vi "Color Steps Control.vi"(7 "Calling VI Ref":refnum<vi>) -> ()   [LabVIEW 2020]
uses:
  <vilib>/Utility/miscctls.llb/LVPointTypeDef.ctl
  Color Steps Type Def/Color Steps Presets Type.ctl
  Color Steps Type Def/Color Steps Step Type.ctl
  Laser Control/Laser Power Control/Laser Power Control Type Defs/Laser Power Ctrl Base Type.ctl
  Color Steps Type Def/Color Steps Notifier Type.ctl
  Color Steps Type Def/Color Step Actions.ctl
  Hardware Configuration/Hardware Configuration Controls/Device Type.ctl
  Hardware Configuration/Hardware Configuration Controls/Device Function.ctl
  Laser Control/Laser Power Control/Laser Power Control Type Defs/Laser Power Ctrl Messenger Actions.ctl
  Device Library/Spinning Disk/Spinning Disk Polymorphic Messenger/Status.vi
  Device Library/Filter Wheels/Polymorphic Filter Wheel Messenger/FW Get Position.vi
  Device Library/Spinning Disk/Spinning Disk Polymorphic Messenger/Set Dichroic Position.vi
  Device Library/Spinning Disk/Spinning Disk Polymorphic Messenger/Set Filter Position.vi
  Device Library/Filter Wheels/Polymorphic Filter Wheel Messenger/FW Set Position.vi
panel:
  in  "Tab Control":enum32{"Step Control", "Setup"}(tab)
  in  "Presets":u16(ring) items=["None"]
  in  "Step":T1(radio)
  in  "Add Step":bool
  in  "Update Step":bool
  in  "Remove Step":bool
  in  "Clear All":bool
  in  "Preset_Name":string
  in  "Step_Name_01":string
  in  "Step_Name_02":string
  in  "Step_Name_03":string
  in  "Step_Name_04":string
  in  "Step_Name_05":string
  in  "Save Preset":bool
  in  "Setup":bool=TRUE
  in  "Quit":bool
  # "Preset Name:"
  # "Step 01 Name:"
  # "Step 04 Name:"
  # "Step 02 Name:"
  # "Step 05 Name:"
  # "Step 03 Name:"
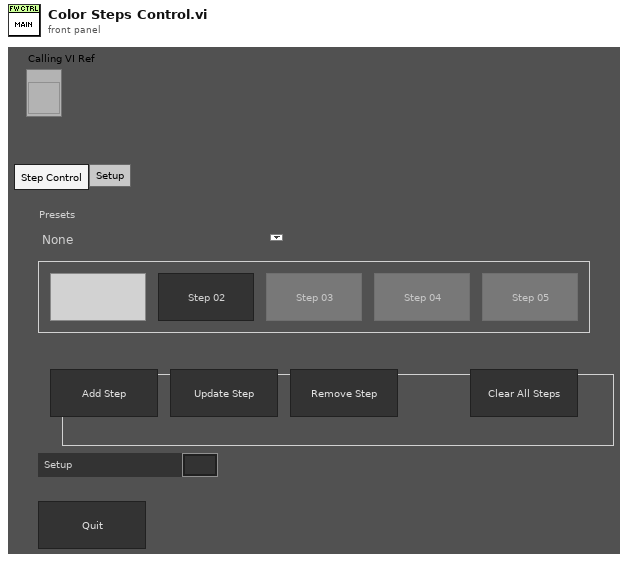
[diagram p1: front panel]
types:
  T1 = enum32{"Step 01", "Step 02", "Step 03", "Step 04", "Step 05"}
  T2 = typedef "Device Function.ctl" = enum16{"Primary", "Secondary", "Overview", "Wide Field Drift Correction", "642 nm Excitation", "560 nm Excitation", "940 nm Excitation", "546 nm Excitation", "488 nm Excitation", "405 nm Excitation", "Objective Drift Correction", "4Pi Objective Lock", "Objective XY", "Objective Z", "Sample XY", "Sample Coarse Z", "Sample Z", "4Pi Lower", "4Pi Upper", "Mojo", "Adj Cavity", "Line Scanning", "Alert"}
  T3 = typedef "Device Type.ctl" = enum16{"AOTF", "Camera", "Deformable Mirror", "Laser", "Microscope Base", "Shutter", "Stage", "Waveform", "FPGA", "Email", "Filter Wheel", "Spinning Disk"}
  T4 = typedef "Color Steps Notifier Type.ctl" = cluster{"Actions":T5, "Set Step":i32, "Current Step":i32, "Last Step?":bool, "Received?":bool, "Preset Index":i32}
  T5 = typedef "Color Step Actions.ctl" = enum16{"Add Step", "Update Step", "Remove Step", "Clear All", "Get Status", "Next Step", "Go To Step", "Save Preset", "Change Preset", "Update Names", "Quit"}
  T6 = typedef "Color Steps Presets Type.ctl" = cluster{"Preset Name":string, "Steps":T7[]}
  T7 = typedef "Color Steps Step Type.ctl" = cluster{"Power Ctrl":T8[], "Filter Wheel Position":i32, "Step Name":string, "Wavelengths":u16[], "SD Dichroic":i32, "SD Filter Wheel":i32}
  T8 = typedef "Laser Power Ctrl Base Type.ctl" = cluster{"Active":bool, "Power":dbl, "Ctrl Mode":u16}
  T9 = enum16{"Always On", "Always Off", "Off While Running"}
  T10 = typedef "LVPointTypeDef.ctl" = cluster{"Horizontal":i16, "Vertical":i16}
  T11 = enum8{"Enabled", "Disabled", "Disabled and Grayed Out"}
  T12 = typedef "LVRectTypeDef.ctl" = cluster{"Left":i16, "Top":i16, "Right":i16, "Bottom":i16}
  T13 = typedef "LVBoundsTypeDef.ctl" = cluster{"Width":u32, "Height":u32}
  T14 = typedef "Laser Power Ctrl Messenger Actions.ctl" = enum16{"All Active On", "All Off", "Adjust Power", "Line On/Off", "Get Status"}
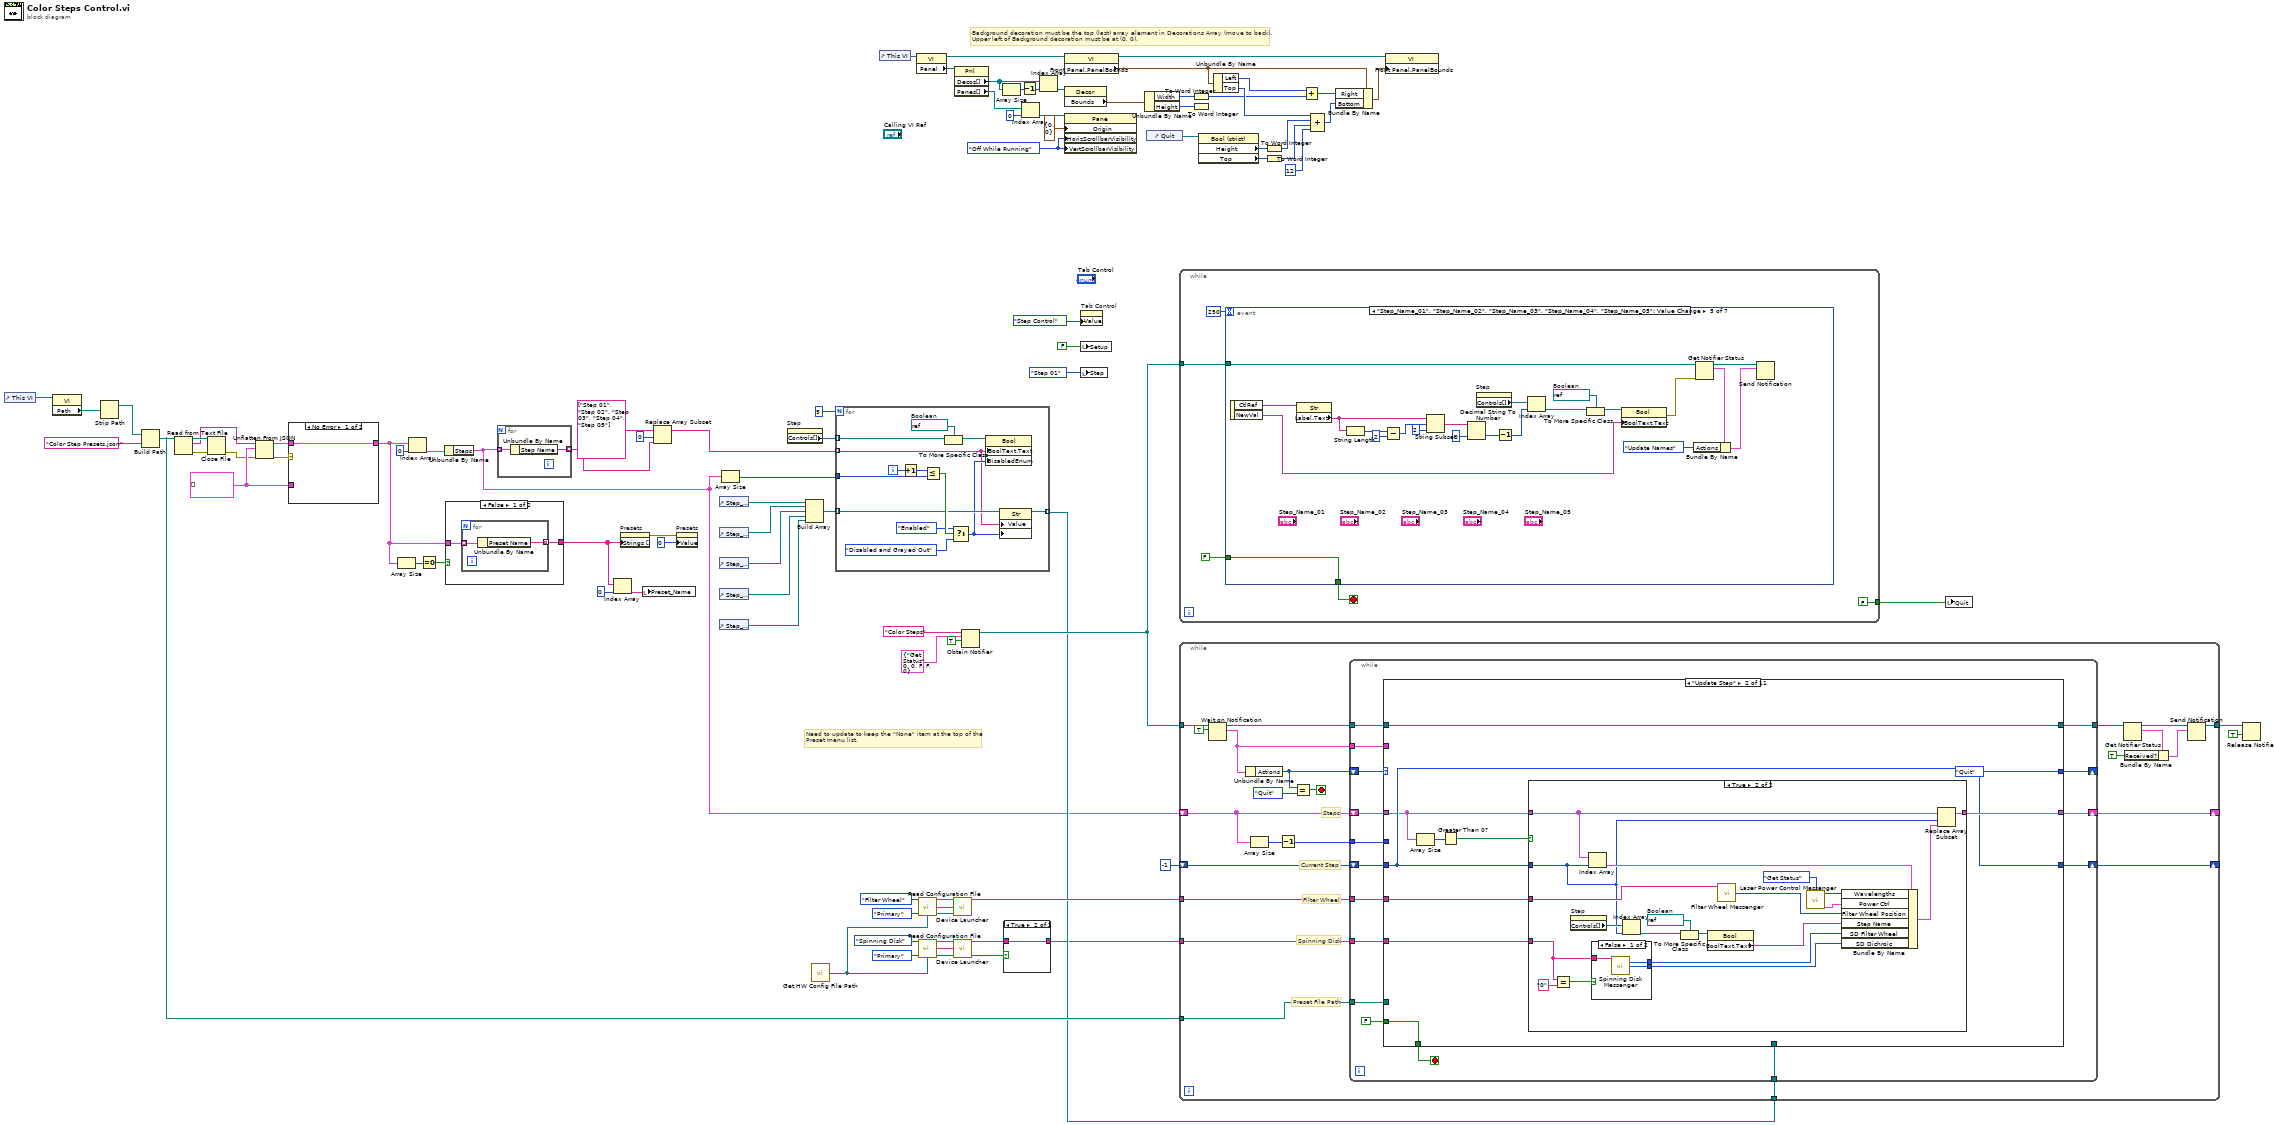
[diagram p0: block diagram]
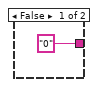
[diagram p2: hidden frame]
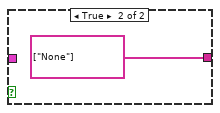
[diagram p3: hidden frame]
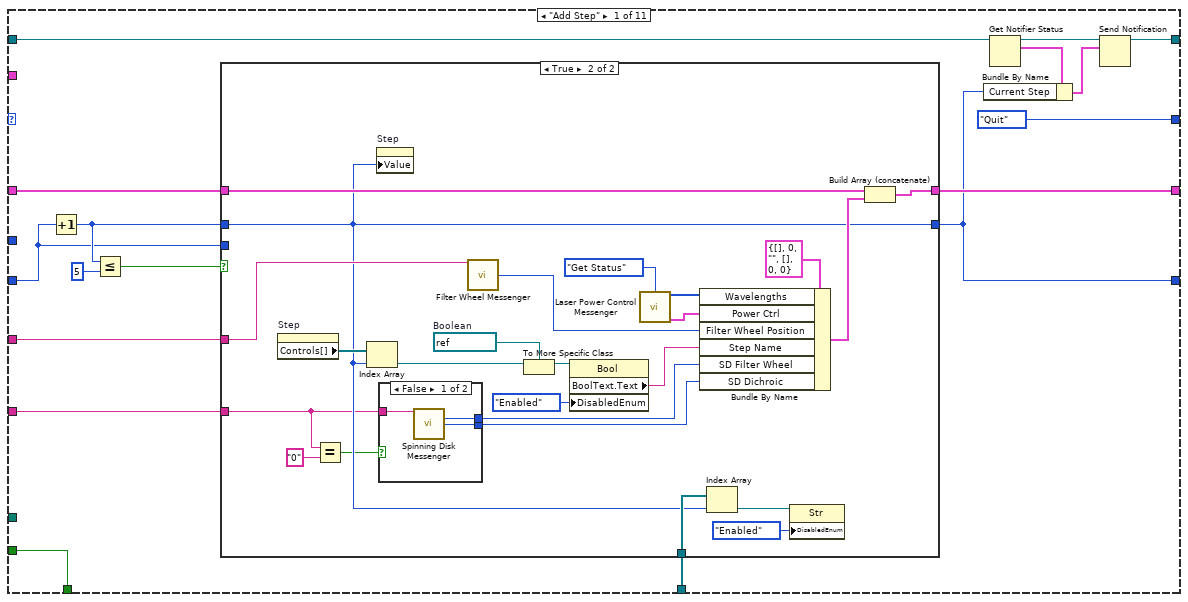
[diagram p4: hidden frame]
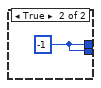
[diagram p6: hidden frame]
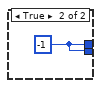
[diagram p8: hidden frame]
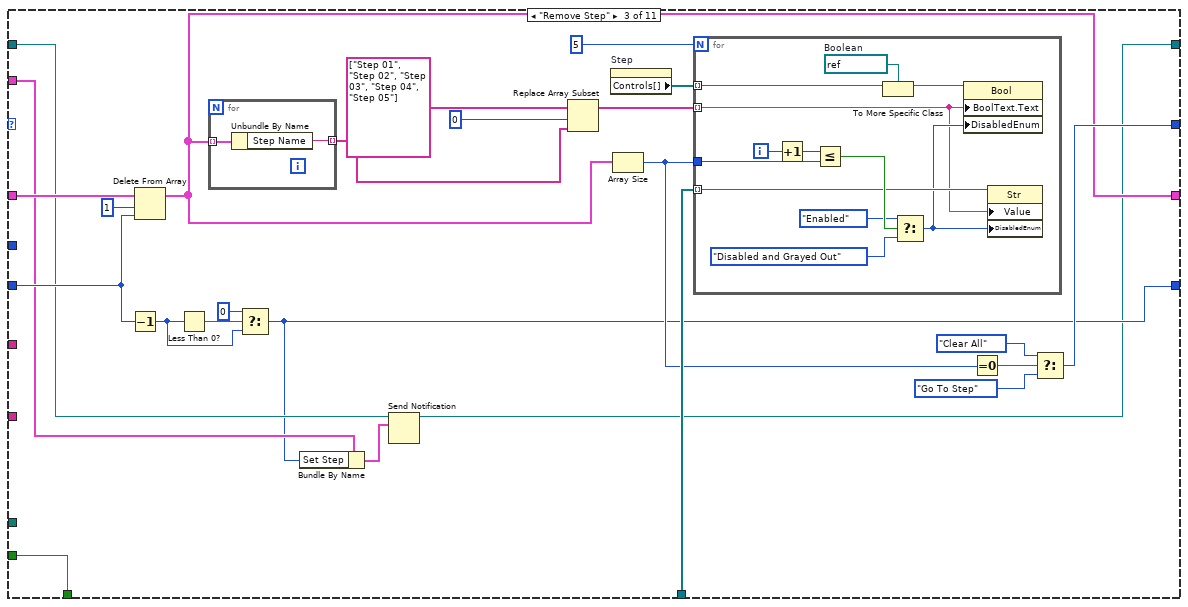
[diagram p9: hidden frame]
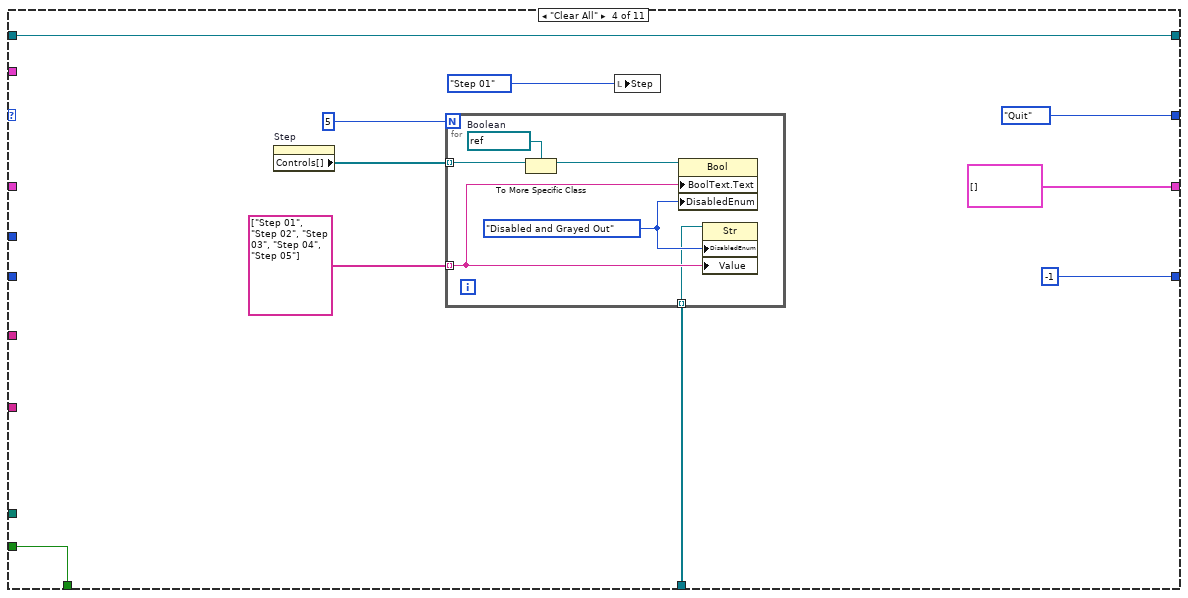
[diagram p10: hidden frame]
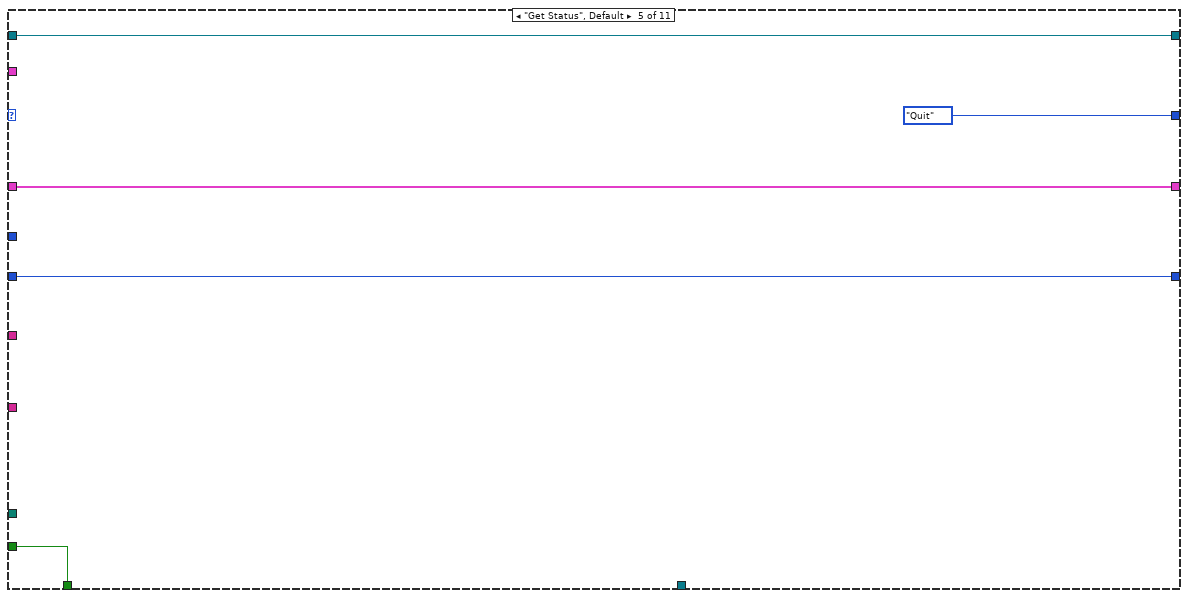
[diagram p11: hidden frame]
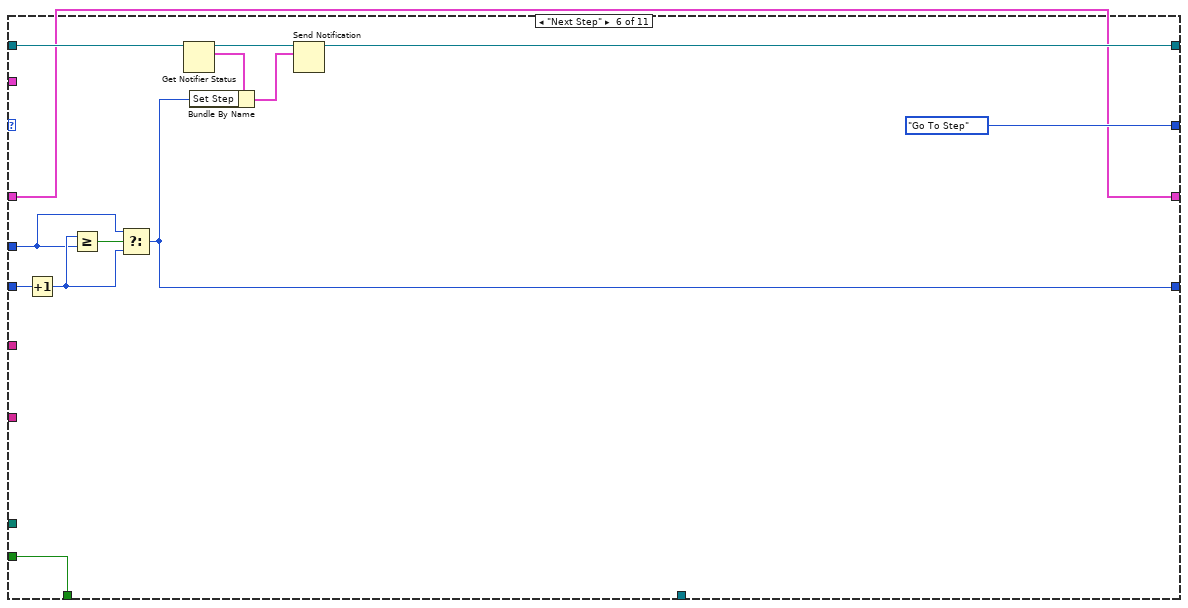
[diagram p12: hidden frame]
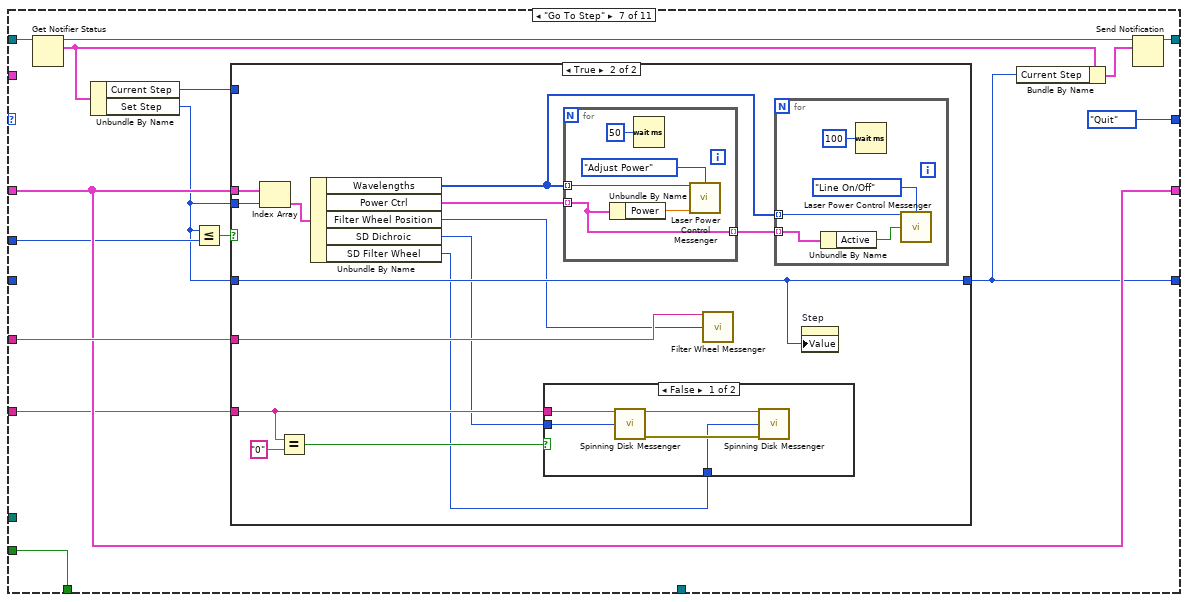
[diagram p13: hidden frame]
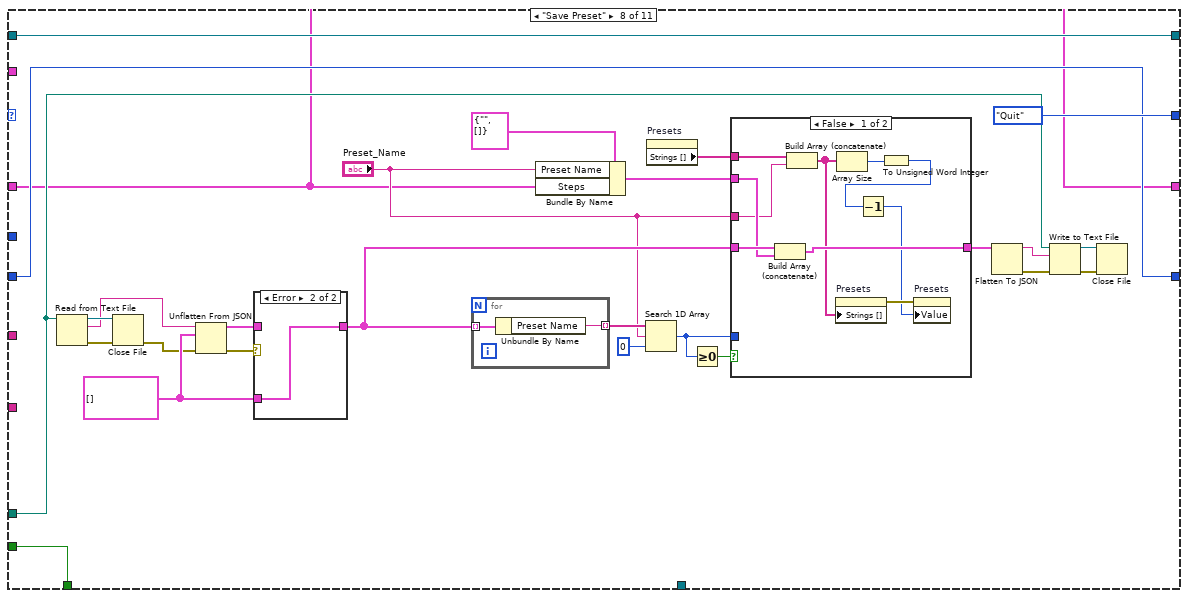
[diagram p16: hidden frame]
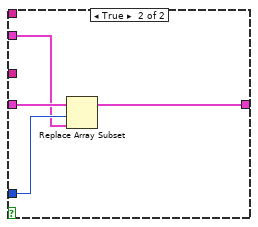
[diagram p17: hidden frame]
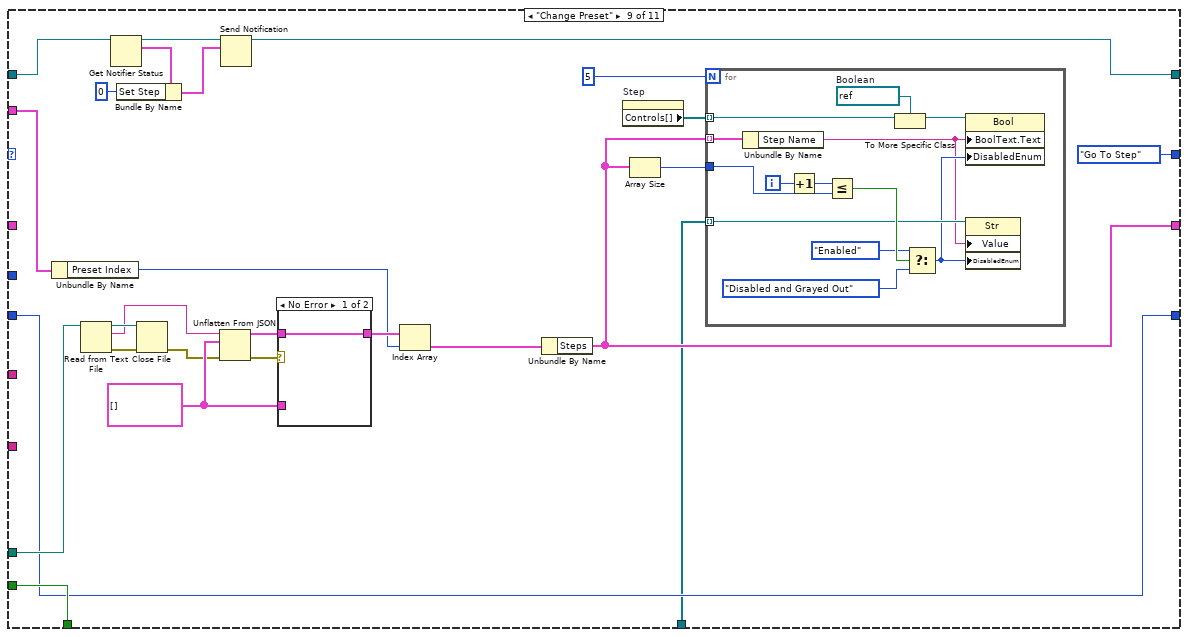
[diagram p19: hidden frame]
diagram:
  w48 = T6[] []
  w75 = T9."Off While Running" ("Vertical Scrollbar Visibility")
  # "Need to update to keep the \"None\" item at the top of the\nPreset menu list."
  # "Background decoration must be the top (last) array element in Decorations Array (move to back).\nUpper left of Background decoration must be at (0, 0)."
  n1 = control-ref of="This VI"() -> (w63:refnum<vi>)
  n2 = property class="VI"(reference=w63) -> ("Path"=w62:path)  [unwired: 1 in, 2 out]
  n3 = Strip Path(path=w62) -> (stripped path=w58:path)  [unwired: 1 out]
  n4 = Build Path(base path=w58, name or relative path="Color Step Presets.json") -> (appended path=w22:path)
  n5 = Read from Text File(file (use dialog)=w22) -> (refnum out=w47:refnum<file>, text=w44:string, error out=w46:errorcluster)  [unwired: 3 in, 1 out]
  n6 = Close File(refnum=w47, error in=w46) -> (error out=w45:errorcluster)  [unwired: 1 out]
  n7 = Unflatten From JSON(JSON string=w44, type and defaults=w48, error in (no error)=w45) -> (value=w59:T6[], error out=w60:errorcluster)  [unwired: 4 in]
  n8 = case shown="No Error" w60 {
    tunnel: w59 -> [w93 _]
    tunnel: w48 -> [_ w94]
    tunnel: [w93 w94] -> w18
    frame No Error {
    }
    frame Error {
    }
  }
  n9 = Array Size(array=w18) -> (size(s)=w17:i32)
  n10 = Index Array(array=w18, index=0) -> (element=w31:T6)
  n11 = Equal To 0?(x=w17) -> (x = 0?=w16:bool)
  n12 = Unbundle By Name(w31) -> ("Steps"=w12:T7[])
  n13 = case shown="False" w16 {
    tunnel: w18 -> [w96 _]
    tunnel: [w95 string[] ["None"]] -> w20
    frame False {
      n14 = for {
        tunnel: w96 -> [w98] mode=indexing
        tunnel: [w97] -> w95 mode=indexing
        n15 = Unbundle By Name(w98) -> ("Preset Name"=w97:string)
      }
    }
    frame True {
    }
  }
  n16 = for {
    tunnel: w12 -> [w101] mode=indexing
    tunnel: [w100] -> w13 mode=indexing
    n17 = Unbundle By Name(w101) -> ("Step Name"=w100:string)
  }
  n18 = Index Array(array=w20, index=0) -> (element=w29:string)
  n19 = property on="Presets" class="Ring (strict)"("Strings []"=w20) -> (error out=w42:errorcluster)  [unwired: 2 in, 1 out]
  n20 = local write "Preset_Name"(w29) -> ()
  n21 = Replace Array Subset(array=string[] ["Step 01", "Step 02", "Step 03", "Step 04", "Step 05"], new element=w13, index=0) -> (w11:string[])
  n22 = property on="Presets" class="Ring (strict)"(error in=w42, "Value"=u16 0) -> ()  [unwired: 1 in, 2 out]
  n23 = control-ref of="Step_Name_01"() -> (w57:refnum<vi>)
  n24 = control-ref of="Step_Name_02"() -> (w53:refnum<vi>)
  n25 = control-ref of="Step_Name_03"() -> (w54:refnum<vi>)
  n26 = control-ref of="Step_Name_04"() -> (w55:refnum<vi>)
  n27 = control-ref of="Step_Name_05"() -> (w56:refnum<vi>)
  n28 = Array Size(array=w12) -> (size(s)=w40:i32)
  n29 = property on="Step" class="RadioBtnsControl (strict)"() -> ("Controls[]"=w51:refnum<vi>[])  [unwired: 2 in, 2 out]
  n30 = Build Array(w57, w53, w54, w55, w56) -> (w43:refnum<vi>[])
  n31 = call "Get HW Config File Path.vi"() -> ("File Path"=w4:path)  [unwired: 14 in, 1 out]
  n32 = for {
    N: 5 -> [_]
    tunnel: [w114] -> w21 mode=indexing
    tunnel: w51 -> [w113] mode=indexing
    tunnel: w43 -> [w105] mode=indexing
    tunnel: w40 -> [w104]
    tunnel: w11 -> [w102] mode=indexing
    i -> [w110]
    w112 = refnum<vi> refnum  # Boolean
    n33 = Increment(x=w110) -> (x+1=w109:i32)
    n34 = Less Or Equal?(x=w109, y=w104) -> (x <= y?=w108:bool)
    n35 = To More Specific Class(target class=w112, reference=w113) -> (specific class reference=w111:refnum<vi>)  [unwired: 1 in, 1 out]
    n36 = Select(t=T11."Enabled" ("Disabled"), s=w108, f=T11."Disabled and Grayed Out") -> (s? t:f=w103:T11)
    n37 = property class="Bool"(reference=w111, "BoolText.Text"=w102, "DisabledEnum"=w103) -> ()  [unwired: 1 in, 2 out]
    n38 = property class="Str"(reference=w105, "Value"=w102, "DisabledEnum"=w103) -> (reference out=w114:refnum<vi>)  [unwired: 1 in, 1 out]
  }
  n39 = control-ref of="This VI"() -> (w67:refnum<vi>)
  n40 = property class="VI"(reference=w67) -> (reference out=w76:refnum<vi>, "Panel"=w68:refnum<vi>)  [unwired: 1 in, 1 out]
  n41 = call "Read Configuration File.vi"("Device Type"=Device_Type."Filter Wheel", "Device Function"=Device_Function."Primary", "Config File Path"=w4) -> ("Unique Notifier Name"=w28:string, "Device Ports/IDs/Channels"=w26:string[], "Device Engine Path"=w27:path)  [unwired: 9 in, 1 out]
  n42 = call "Read Configuration File.vi"("Device Type"=Device_Type."Spinning Disk", "Device Function"=Device_Function."Primary", "Config File Path"=w4) -> ("Unique Notifier Name"=w5:string, "Device Ports/IDs/Channels"=w7:string[], "Device Engine Path"=w6:path)  [unwired: 9 in, 1 out]
  n43 = call "Device Launcher.vi"("Notifier Name"=w28, "Device Ports/IDs/Channels"=w26, "Device Engine Path"=w27) -> ("Notifier Name"=w23:string)  [unwired: 11 in, 1 out]
  n44 = call "Device Launcher.vi"("Notifier Name"=w5, "Device Ports/IDs/Channels"=w7, "Device Engine Path"=w6) -> ("Notifier Name"=w2:string, "Running?"=w3:bool)  [unwired: 11 in]
  n45 = property class="Pnl"(reference=w68) -> ("Decos[]"=w66:refnum<vi>[], "Panes[]"=w72:refnum<vi>[])  [unwired: 1 in, 2 out]
  n46 = Obtain Notifier(name (unnamed)="Color Steps", notification data type=T4 {"Actions"=enum."Get Status", "Set Step"=0, "Current Step"=0, "Last Step?"=FALSE, "Received?"=FALSE, "Preset Index"=0} ("Color Steps Note Type"), create if not found? (T)=TRUE) -> (notifier out=w35:refnum<notifier>)  [unwired: 1 in, 2 out]
  n47 = Array Size(array=w66) -> (size(s)=w64:i32)
  n48 = case shown="True" w3 {
    tunnel: w2 -> [_ w116]
    tunnel: ["0" w116] -> w1
    frame False {
    }
    frame True {
    }
  }
  n49 = Decrement(x=w64) -> (x-1=w65:i32)
  n50 = Index Array(array=w72, index=0) -> (element=w71:refnum<vi>)
  n51 = Index Array(array=w66, index=w65) -> (element=w74:refnum<vi>)
  n52 = property class="VI"(reference=w76) -> (reference out=w78:refnum<vi>, "Front Panel.PanelBounds"=w79:T12)  [unwired: 1 in, 1 out]
  n53 = property class="Decor"(reference=w74) -> ("Bounds"=w77:T13)  [unwired: 1 in, 2 out]
  n54 = property class="Pane"(reference=w71, "Origin"=T10 {"Horizontal"=0, "Vertical"=0}, "HorizScrollbarVisibility"=w75, "VertScrollbarVisibility"=w75) -> ()  [unwired: 1 in, 2 out]
  n55 = property on="Tab Control" class="TabCtl (strict)"("Value"=enum32{"Step Control", "Setup"}."Step Control" ("Tab Control")) -> ()  [unwired: 2 in, 2 out]
  n56 = local write "Setup"(FALSE ("Filter Wheel Setup")) -> ()
  n57 = local write "Step"(T1."Step 01" ("Step")) -> ()
  n58 = Unbundle By Name(w77) -> ("Width"=w82:u32, "Height"=w85:u32)
  n59 = control-ref of="Quit"() -> (w69:refnum<vi>)
  n60 = while {
    tunnel: w35 -> [w118]
    tunnel: [FALSE] -> w10
    stop <- w120 stop-if-true
    n61 = event shown="[4] \"Step_Name_01\", \"Step_Name_02\", \"Step_Name_03\", \"Step_Name_04\", \"Step_Name_05\": Value Change" {
      selector: _ -> [_ _ _ _ _ _ _]
      dyn-events: _ -> [_ _ _ _ _ _ _]
      timeout: 250 -> [_ _ _ _ _ _ _]
      tunnel: FALSE -> [_ w132 w140 w151 w173 w181 _]
      tunnel: [w122 w132 w140 w151 w173 w181 w187] -> w120
      tunnel: w118 -> [w124 w131 w134 _ w153 w176 w182]
      event Timeout {
        n62 = event-data() -> ()  [unwired: 1 in, 3 out]
        n63 = Get Notifier Status(notifier=w124) -> (error out=w123:errorcluster)  [unwired: 1 in, 4 out]
        n64 = Unbundle By Name(w123) -> ("status"=w122:bool)
      }
      event "Step": Value Change {
        n65 = event-data() -> ("NewVal"=w126:T1)  [unwired: 1 in]
        n66 = To Long Integer(number=w126) -> (32bit integer=w125:i32)
        n67 = Get Notifier Status(notifier=w131) -> (notifier out=w130:refnum<notifier>, current notification=w129:T4)  [unwired: 1 in, 3 out]
        n68 = Bundle By Name(cluster=w129, "Actions"=Color_Step_Actions."Go To Step", "Set Step"=w125) -> (w127:T4)
        n69 = Send Notification(notification=w127, notifier=w130) -> ()  [unwired: 1 in, 2 out]
      }
      event "Add Step", "Update Step", "Remove Step", "Clear All", "Save Preset": Value Change {
        n70 = event-data() -> ("CtlRef"=w139:refnum<vi>)  [unwired: 1 in]
        n71 = property class="Bool"(reference=w139) -> ("Label.Text"=w138:string)  [unwired: 1 in, 2 out]
        n72 = case shown="\"Add Step\"" w138 {
          tunnel: [Color_Step_Actions."Get Status" ("Actions") Color_Step_Actions."Add Step" ("Actions") Color_Step_Actions."Update Step" ("Actions") Color_Step_Actions."Remove Step" ("Actions") Color_Step_Actions."Clear All" ("Actions") Color_Step_Actions."Save Preset" ("Actions")] -> w133
          frame Default {
          }
          frame "Add Step" {
          }
          frame "Update Step" {
          }
          frame "Remove Step" {
          }
          frame "Clear All" {
          }
          frame "Save Preset" {
          }
        }
        n73 = Get Notifier Status(notifier=w134) -> (notifier out=w137:refnum<notifier>, current notification=w136:T4)  [unwired: 1 in, 3 out]
        n74 = Bundle By Name(cluster=w136, "Actions"=w133) -> (w135:T4)
        n75 = Send Notification(notification=w135, notifier=w137) -> ()  [unwired: 1 in, 2 out]
      }
      event "Setup": Value Change {
        n76 = event-data() -> ("NewVal"=w150:bool)  [unwired: 1 in]
        n77 = Select(t=enum32{"Step Control", "Setup"}."Setup" ("Tab Control"), s=w150, f=enum32{"Step Control", "Setup"}."Step Control" ("Tab Control")) -> (s? t:f=w147:enum32{"Step Control", "Setup"})
        n78 = property on="Tab Control" class="TabCtl (strict)"("Value"=w147) -> ()  [unwired: 2 in, 2 out]
      }
      event "Step_Name_01", "Step_Name_02", "Step_Name_03", "Step_Name_04", "Step_Name_05": Value Change {
        w172 = refnum<vi> refnum  # Boolean
        n79 = event-data() -> ("CtlRef"=w159:refnum<vi>, "NewVal"=w158:string)  [unwired: 1 in]
        n80 = property class="Str"(reference=w159) -> ("Label.Text"=w170:string)  [unwired: 1 in, 2 out]
        n81 = String Length(string=w170) -> (length=w169:i32)
        n82 = Subtract(x=w169, y=2) -> (x-y=w167:i32)
        n83 = String Subset(string=w170, offset (0)=w167, length (rest)=2 ("length (rest)")) -> (substring=w166:string)
        n84 = Decimal String To Number(string=w166, default (0L)=0 ("default (0 I32)")) -> (number=w163:i32)  [unwired: 1 in, 1 out]
        n85 = property on="Step" class="RadioBtnsControl (strict)"() -> ("Controls[]"=w164:refnum<vi>[])  [unwired: 2 in, 2 out]
        n86 = Decrement(x=w163) -> (x-1=w160:i32)
        n87 = Index Array(array=w164, index=w160) -> (element=w162:refnum<vi>)
        n88 = To More Specific Class(target class=w172, reference=w162) -> (specific class reference=w161:refnum<vi>)  [unwired: 1 in, 1 out]
        n89 = property class="Bool"(reference=w161, "BoolText.Text"=w158) -> (error out=w152:errorcluster)  [unwired: 1 in, 1 out]
        n90 = Get Notifier Status(notifier=w153, error in (no error)=w152) -> (notifier out=w157:refnum<notifier>, current notification=w156:T4)  [unwired: 3 out]
        n91 = Bundle By Name(cluster=w156, "Actions"=Color_Step_Actions."Update Names") -> (w154:T4)
        n92 = Send Notification(notification=w154, notifier=w157) -> ()  [unwired: 1 in, 2 out]
      }
      event "Presets": Value Change {
        n93 = event-data() -> ("NewVal"=w175:u16)  [unwired: 1 in]
        n94 = To Long Integer(number=w175) -> (32bit integer=w174:i32)
        n95 = Get Notifier Status(notifier=w176) -> (notifier out=w180:refnum<notifier>, current notification=w179:T4)  [unwired: 1 in, 3 out]
        n96 = Bundle By Name(cluster=w179, "Actions"=Color_Step_Actions."Change Preset", "Preset Index"=w174) -> (w177:T4)
        n97 = Send Notification(notification=w177, notifier=w180) -> ()  [unwired: 1 in, 2 out]
      }
      event "Quit": Value Change {
        n98 = event-data() -> ("NewVal"=w187:bool)  [unwired: 1 in]
        n99 = Get Notifier Status(notifier=w182) -> (notifier out=w186:refnum<notifier>, current notification=w185:T4)  [unwired: 1 in, 3 out]
        n100 = Bundle By Name(cluster=w185, "Actions"=Color_Step_Actions."Quit") -> (w183:T4)
        n101 = Send Notification(notification=w183, notifier=w186) -> ()  [unwired: 1 in, 2 out]
      }
    }
  }
  n102 = while {
    tunnel: w35 -> [w210]
    shift-right: [w196] -> _
    shift-left: w12 -> [w203]
    tunnel: [w189] -> w34
    shift-right: [w199] -> _
    shift-left: -1 -> [w204]
    tunnel: w23 -> [w200]
    tunnel: w22 -> [w198]
    tunnel: w21 -> [w195]
    tunnel: w1 -> [w188]
    stop <- w207 stop-if-true
    # "Spinning Disk"
    # "Preset File Path"
    # "Filter Wheel"
    # "Steps"
    # "Current Step"
    n103 = Wait on Notification(notifier=w210, ignore previous (F)=TRUE) -> (notifier out=w206:refnum<notifier>, notification=w197:T4)  [unwired: 2 in, 2 out]
    n104 = Unbundle By Name(w197) -> ("Actions"=w205:T5)
    n105 = Array Size(array=w203) -> (size(s)=w202:i32)
    n106 = Decrement(x=w202) -> (x-1=w201:i32)
    n107 = Equal?(x=w205, y=Color_Step_Actions."Quit") -> (x = y?=w207:bool)
    n108 = while {
      tunnel: w206 -> [w226]
      shift-right: [w218] -> _
      shift-left: w205 -> [w225]
      shift-right: [w213] -> w199
      shift-left: w204 -> [w220]
      shift-right: [w215] -> w196
      shift-left: w203 -> [w221]
      tunnel: w201 -> [w222]
      tunnel: w200 -> [w219]
      tunnel: w198 -> [w217]
      tunnel: w197 -> [w216]
      tunnel: w195 -> [w214]
      tunnel: [w212] -> w190
      tunnel: w188 -> [w211]
      stop <- w223 stop-if-true
      n109 = case shown="\"Update Step\"" w225 {
        tunnel: w226 -> [w235 w278 w313 w356 w367 w376 w385 w430 w474 w519 w535]
        tunnel: FALSE -> [w243 w283 w333 w357 w368 w381 w396 w453 w497 w520 _]
        tunnel: [w243 w283 w333 w357 w368 w381 w396 w453 w497 w520 TRUE] -> w223
        tunnel: [w234 w278 w310 w356 w367 w375 w393 w430 w472 w519 w534] -> w212
        tunnel: w222 -> [_ _ _ _ _ w371 w390 _ _ _ w533]
        tunnel: w221 -> [w242 w277 w332 _ w364 w370 w391 w427 _ w516 w531]
        tunnel: w220 -> [w229 w280 w330 _ w366 w380 _ w432 w484 w513 w532]
        tunnel: w219 -> [w239 w282 _ _ _ _ w395 _ _ _ _]
        tunnel: [w233 w280 w311 -1 ("Set Step") w366 w369 w386 w432 w484 w513 w532] -> w213
        tunnel: [Color_Step_Actions."Quit" ("y") Color_Step_Actions."Quit" ("y") w318 Color_Step_Actions."Quit" ("y") Color_Step_Actions."Quit" ("y") Color_Step_Actions."Go To Step" ("y") Color_Step_Actions."Quit" ("y") Color_Step_Actions."Quit" ("y") Color_Step_Actions."Go To Step" ("y") Color_Step_Actions."Quit" ("y") Color_Step_Actions."Quit" ("y")] -> w218
        tunnel: w217 -> [_ _ _ _ _ _ _ w435 w489 _ _]
        tunnel: w216 -> [_ _ w314 _ _ _ _ _ w488 _ _]
        tunnel: [w240 w281 w317 T7[] [] ("Steps") w364 w370 w391 w427 w480 w517 w531] -> w215
        tunnel: w214 -> [w228 _ w325 w350 _ _ _ _ w478 _ _]
        tunnel: w211 -> [w227 w274 _ _ _ _ w382 _ _ _ _]
        frame "Add Step" {
          n110 = Increment(x=w229) -> (x+1=w231:i32)
          n111 = Less Or Equal?(x=w231, y=5) -> (x <= y?=w232:bool)
          n112 = case shown="True" w232 {
            tunnel: w242 -> [w245 w269]
            tunnel: [w245 w268] -> w240
            tunnel: w239 -> [_ w259]
            tunnel: w231 -> [_ w252]
            tunnel: [w244 w252] -> w233
            tunnel: w229 -> [w244 _]
            tunnel: w228 -> [_ w255]
            tunnel: w227 -> [_ w250]
            frame False {
            }
            frame True {
              w266 = refnum<vi> refnum  # Boolean
              n113 = property on="Step" class="RadioBtnsControl (strict)"() -> ("Controls[]"=w267:refnum<vi>[])  [unwired: 2 in, 2 out]
              n114 = Equal?(x=w250, y="0") -> (x = y?=w249:bool)
              n115 = Index Array(array=w267, index=w252) -> (element=w265:refnum<vi>)
              n116 = property on="Step" class="RadioBtnsControl (strict)"("Value"=w252) -> ()  [unwired: 2 in, 2 out]
              n117 = case shown="False" w249 {
                tunnel: w250 -> [w272 _]
                tunnel: [w271 w273] -> w247
                tunnel: [w270 w273] -> w248
                frame False {
                  n118 = call-poly "Spinning Disk Messenger.vi"("Notifier Name"=w272) -> ("Filter Wheel"=w270:i32, "Dichroic"=w271:i32)  [unwired: 9 in, 4 out]
                }
                frame True {
                  w273 = -1 ("Filter Wheel")
                }
              }
              n119 = call-poly "Filter Wheel Messenger.vi"("Notifier Name In"=w259) -> ("Position"=w246:i32)  [unwired: 12 in, 2 out]
              n120 = To More Specific Class(target class=w266, reference=w265) -> (specific class reference=w264:refnum<vi>)  [unwired: 1 in, 1 out]
              n121 = property class="Bool"(reference=w264, "DisabledEnum"=T11."Enabled" ("Disabled")) -> ("BoolText.Text"=w263:string)  [unwired: 1 in, 2 out]
              n122 = call "Laser Power Control Messenger.vi"("Power Ctrl Actions"=Laser_Power_Ctrl_Messenger_Actions."Get Status") -> ("Wavelengths"=w261:u16[], "Power Status"=w260:T8[])  [unwired: 13 in]
              n123 = Bundle By Name(cluster=T7 {"Power Ctrl"=[], "Filter Wheel Position"=0, "Step Name"="", "Wavelengths"=[], "SD Dichroic"=0, "SD Filter Wheel"=0} ("Step"), "Wavelengths"=w261, "Power Ctrl"=w260, "Filter Wheel Position"=w246, "Step Name"=w263, "SD Filter Wheel"=w248, "SD Dichroic"=w247) -> (w257:T7)
              n124 = Index Array(array=w255, index=w252) -> (element=w254:refnum<vi>)
              n125 = property class="Str"(reference=w254, "DisabledEnum"=T11."Enabled" ("Disabled")) -> ()  [unwired: 1 in, 2 out]
              n126 = Build Array (concatenate)(w269, w257) -> (w268:T7[])
            }
          }
          n127 = Get Notifier Status(notifier=w235) -> (notifier out=w236:refnum<notifier>, current notification=w237:T4)  [unwired: 1 in, 3 out]
          n128 = Bundle By Name(cluster=w237, "Current Step"=w233) -> (w238:T4)
          n129 = Send Notification(notification=w238, notifier=w236) -> (notifier out=w234:refnum<notifier>)  [unwired: 1 in, 1 out]
        }
        frame "Update Step" {
          n130 = Array Size(array=w277) -> (size(s)=w276:i32)
          n131 = Greater Than 0?(x=w276) -> (x > 0?=w275:bool)
          n132 = case shown="True" w275 {
            tunnel: w282 -> [_ w297]
            tunnel: [w284 w292] -> w281
            tunnel: w280 -> [_ w291]
            tunnel: w277 -> [w284 w290]
            tunnel: w274 -> [_ w287]
            frame False {
            }
            frame True {
              w301 = refnum<vi> refnum  # Boolean
              n133 = Equal?(x=w287, y="0") -> (x = y?=w289:bool)
              n134 = property on="Step" class="RadioBtnsControl (strict)"() -> ("Controls[]"=w302:refnum<vi>[])  [unwired: 2 in, 2 out]
              n135 = Index Array(array=w290, index=w291) -> (element=w304:T7)
              n136 = case shown="False" w289 {
                tunnel: w287 -> [w307 _]
                tunnel: [w306 w308] -> w285
                tunnel: [w305 w308] -> w286
                frame False {
                  n137 = call-poly "Spinning Disk Messenger.vi"("Notifier Name"=w307) -> ("Filter Wheel"=w305:i32, "Dichroic"=w306:i32)  [unwired: 9 in, 4 out]
                }
                frame True {
                  w308 = -1 ("Filter Wheel")
                }
              }
              n138 = Index Array(array=w302, index=w291) -> (element=w300:refnum<vi>)
              n139 = To More Specific Class(target class=w301, reference=w300) -> (specific class reference=w299:refnum<vi>)  [unwired: 1 in, 1 out]
              n140 = property class="Bool"(reference=w299) -> ("BoolText.Text"=w298:string)  [unwired: 1 in, 2 out]
              n141 = call-poly "Filter Wheel Messenger.vi"("Notifier Name In"=w297) -> ("Position"=w296:i32)  [unwired: 12 in, 2 out]
              n142 = call "Laser Power Control Messenger.vi"("Power Ctrl Actions"=Laser_Power_Ctrl_Messenger_Actions."Get Status") -> ("Wavelengths"=w294:u16[], "Power Status"=w293:T8[])  [unwired: 13 in]
              n143 = Bundle By Name(cluster=w304, "Wavelengths"=w294, "Power Ctrl"=w293, "Filter Wheel Position"=w296, "Step Name"=w298, "SD Filter Wheel"=w286, "SD Dichroic"=w285) -> (w303:T7)
              n144 = Replace Array Subset(array=w290, new element=w303, index=w291) -> (w292:T7[])
            }
          }
        }
        frame "Remove Step" {
          n145 = Decrement(x=w330) -> (x-1=w329:i32)
          n146 = Delete From Array(array=w332, length=1, index=w330) -> (array with subset deleted=w317:T7[])  [unwired: 1 out]
          n147 = Less Than 0?(x=w329) -> (x < 0?=w319:bool)
          n148 = for {
            tunnel: w317 -> [w335] mode=indexing
            tunnel: [w334] -> w322 mode=indexing
            n149 = Unbundle By Name(w335) -> ("Step Name"=w334:string)
          }
          n150 = Select(t=0, s=w319, f=w329) -> (s? t:f=w311:i32)
          n151 = Bundle By Name(cluster=w314, "Set Step"=w311) -> (w312:T4)
          n152 = Send Notification(notification=w312, notifier=w313) -> (notifier out=w310:refnum<notifier>)  [unwired: 1 in, 1 out]
          n153 = Replace Array Subset(array=string[] ["Step 01", "Step 02", "Step 03", "Step 04", "Step 05"], new element=w322, index=0) -> (w321:string[])
          n154 = property on="Step" class="RadioBtnsControl (strict)"() -> ("Controls[]"=w326:refnum<vi>[])  [unwired: 2 in, 2 out]
          n155 = Array Size(array=w317) -> (size(s)=w316:i32)
          n156 = for {
            N: 5 -> [_]
            tunnel: w326 -> [w347] mode=indexing
            tunnel: w325 -> [w339] mode=indexing
            tunnel: w316 -> [w338]
            tunnel: w321 -> [w336] mode=indexing
            i -> [w344]
            w346 = refnum<vi> refnum  # Boolean
            n157 = Increment(x=w344) -> (x+1=w343:i32)
            n158 = Less Or Equal?(x=w343, y=w338) -> (x <= y?=w342:bool)
            n159 = To More Specific Class(target class=w346, reference=w347) -> (specific class reference=w345:refnum<vi>)  [unwired: 1 in, 1 out]
            n160 = Select(t=T11."Enabled" ("Disabled"), s=w342, f=T11."Disabled and Grayed Out") -> (s? t:f=w337:T11)
            n161 = property class="Bool"(reference=w345, "BoolText.Text"=w336, "DisabledEnum"=w337) -> ()  [unwired: 1 in, 2 out]
            n162 = property class="Str"(reference=w339, "Value"=w336, "DisabledEnum"=w337) -> ()  [unwired: 1 in, 2 out]
          }
          n163 = Equal To 0?(x=w316) -> (x = 0?=w315:bool)
          n164 = Select(t=Color_Step_Actions."Clear All" ("y"), s=w315, f=Color_Step_Actions."Go To Step" ("y")) -> (s? t:f=w318:T5)
        }
        frame "Clear All" {
          n165 = property on="Step" class="RadioBtnsControl (strict)"() -> ("Controls[]"=w352:refnum<vi>[])  [unwired: 2 in, 2 out]
          n166 = for {
            N: 5 -> [_]
            tunnel: w352 -> [w363] mode=indexing
            tunnel: string[] ["Step 01", "Step 02", "Step 03", "Step 04", "Step 05"] -> [w359] mode=indexing
            tunnel: w350 -> [w358] mode=indexing
            w360 = T11."Disabled and Grayed Out" ("f")
            w362 = refnum<vi> refnum  # Boolean
            n167 = To More Specific Class(target class=w362, reference=w363) -> (specific class reference=w361:refnum<vi>)  [unwired: 1 in, 1 out]
            n168 = property class="Bool"(reference=w361, "BoolText.Text"=w359, "DisabledEnum"=w360) -> ()  [unwired: 1 in, 2 out]
            n169 = property class="Str"(reference=w358, "DisabledEnum"=w360, "Value"=w359) -> ()  [unwired: 1 in, 2 out]
          }
          n170 = local write "Step"(T1."Step 01" ("Step")) -> ()
        }
        frame "Get Status", Default {
        }
        frame "Next Step" {
          n171 = Increment(x=w380) -> (x+1=w373:i32)
          n172 = Greater Or Equal?(x=w373, y=w371) -> (x >= y?=w372:bool)
          n173 = Select(t=w371, s=w372, f=w373) -> (s? t:f=w369:i32)
          n174 = Get Notifier Status(notifier=w376) -> (notifier out=w377:refnum<notifier>, current notification=w378:T4)  [unwired: 1 in, 3 out]
          n175 = Bundle By Name(cluster=w378, "Set Step"=w369) -> (w379:T4)
          n176 = Send Notification(notification=w379, notifier=w377) -> (notifier out=w375:refnum<notifier>)  [unwired: 1 in, 1 out]
        }
        frame "Go To Step" {
          n177 = Get Notifier Status(notifier=w385) -> (notifier out=w384:refnum<notifier>, current notification=w383:T4)  [unwired: 1 in, 3 out]
          n178 = Unbundle By Name(w383) -> ("Current Step"=w387:i32, "Set Step"=w388:i32)
          n179 = Less Or Equal?(x=w388, y=w390) -> (x <= y?=w389:bool)
          n180 = case shown="True" w389 {
            tunnel: w395 -> [_ w407]
            tunnel: w388 -> [_ w406]
            tunnel: w391 -> [_ w405]
            tunnel: w388 -> [_ w404]
            tunnel: [w397 w404] -> w386
            tunnel: w387 -> [w397 _]
            tunnel: w382 -> [_ w401]
            frame False {
            }
            frame True {
              n181 = Index Array(array=w405, index=w406) -> (element=w408:T7)
              n182 = Equal?(x=w401, y="0") -> (x = y?=w402:bool)
              n183 = Unbundle By Name(w408) -> ("Wavelengths"=w411:u16[], "Power Ctrl"=w409:T8[], "Filter Wheel Position"=w398:i32, "SD Dichroic"=w399:i32, "SD Filter Wheel"=w400:i32)
              n184 = case shown="False" w402 {
                tunnel: w401 -> [w416 _]
                tunnel: w400 -> [w413 _]
                tunnel: w399 -> [w412 _]
                frame False {
                  n185 = call-poly "Spinning Disk Messenger.vi"("Notifier Name"=w416, "Dichroic Position"=w412) -> ("Notifier Name Dup"=w415:string, "Error Out"=w414:errorcluster)  [unwired: 10 in, 2 out]
                  n186 = call-poly "Spinning Disk Messenger.vi"("Notifier Name"=w415, "Filter Position"=w413, "Error In"=w414) -> ()  [unwired: 9 in, 4 out]
                }
                frame True {
                }
              }
              n187 = for {
                tunnel: w409 -> [w423] mode=indexing
                tunnel: w411 -> [w424] mode=indexing
                tunnel: [w423] -> w410 mode=indexing
                n188 = Unbundle By Name(w423) -> ("Power"=w425:dbl)
                n189 = Wait (ms)(milliseconds to wait=u32 50) -> ()  [unwired: 1 out]
                n190 = call "Laser Power Control Messenger.vi"("Wavelength (nm)"=w424, "Power Ctrl Actions"=Laser_Power_Ctrl_Messenger_Actions."Adjust Power", "Power"=w425) -> ()  [unwired: 11 in, 2 out]
              }
              n191 = call-poly "Filter Wheel Messenger.vi"("Notifier Name In"=w407, "Position"=w398) -> ()  [unwired: 12 in, 2 out]
              n192 = for {
                tunnel: w410 -> [w419] mode=indexing
                tunnel: w411 -> [w420] mode=indexing
                n193 = Unbundle By Name(w419) -> ("Active"=w418:bool)
                n194 = Wait (ms)(milliseconds to wait=u32 100) -> ()  [unwired: 1 out]
                n195 = call "Laser Power Control Messenger.vi"("Wavelength (nm)"=w420, "Power Ctrl Actions"=Laser_Power_Ctrl_Messenger_Actions."Line On/Off", "Line On/Off"=w418) -> ()  [unwired: 11 in, 2 out]
              }
              n196 = property on="Step" class="RadioBtnsControl (strict)"("Value"=w404) -> ()  [unwired: 2 in, 2 out]
            }
          }
          n197 = Bundle By Name(cluster=w383, "Current Step"=w386) -> (w394:T4)
          n198 = Send Notification(notification=w394, notifier=w384) -> (notifier out=w393:refnum<notifier>)  [unwired: 1 in, 1 out]
        }
        frame "Save Preset" {
          w449 = T6[] []
          n199 = Read from Text File(file (use dialog)=w435) -> (refnum out=w448:refnum<file>, text=w445:string, error out=w447:errorcluster)  [unwired: 3 in, 1 out]
          n200 = Close File(refnum=w448, error in=w447) -> (error out=w446:errorcluster)  [unwired: 1 out]
          n201 = Unflatten From JSON(JSON string=w445, type and defaults=w449, error in (no error)=w446) -> (value=w450:T6[], error out=w451:errorcluster)  [unwired: 4 in]
          n202 = case shown="Error" w451 {
            tunnel: w450 -> [w470 _]
            tunnel: w449 -> [_ w471]
            tunnel: [w470 w471] -> w441
            frame No Error {
            }
            frame Error {
            }
          }
          n203 = for {
            tunnel: w441 -> [w469] mode=indexing
            tunnel: [w468] -> w444 mode=indexing
            n204 = Unbundle By Name(w469) -> ("Preset Name"=w468:string)
          }
          n205 = Bundle By Name(cluster=T6 {"Preset Name"="", "Steps"=[]} ("Presets"), "Preset Name"="Preset_Name", "Steps"=w427) -> (w439:T6)
          n206 = Search 1D Array(1D array=w444, element="Preset_Name", start index (0)=0) -> (index of element=w442:i32)
          n207 = property on="Presets" class="Ring (strict)"() -> ("Strings []"=w429:string[])  [unwired: 2 in, 2 out]
          n208 = Greater Or Equal To 0?(x=w442) -> (x >= 0?=w443:bool)
          n209 = case shown="False" w443 {
            tunnel: w442 -> [_ w466]
            tunnel: w441 -> [w463 w467]
            tunnel: w439 -> [w462 w464]
            tunnel: [w461 w465] -> w438
            tunnel: w429 -> [w460 _]
            tunnel: "Preset_Name" -> [w459 _]
            frame False {
              n210 = Build Array (concatenate)(w463, w462) -> (w461:T6[])
              n211 = Build Array (concatenate)(w460, w459) -> (w457:string[])
              n212 = property on="Presets" class="Ring (strict)"("Strings []"=w457) -> (error out=w458:errorcluster)  [unwired: 2 in, 1 out]
              n213 = Array Size(array=w457) -> (size(s)=w456:i32)
              n214 = To Unsigned Word Integer(number=w456) -> (unsigned 16bit integer=w455:u16)
              n215 = Decrement(x=w455) -> (x-1=w454:u16)
              n216 = property on="Presets" class="Ring (strict)"(error in=w458, "Value"=w454) -> ()  [unwired: 1 in, 2 out]
            }
            frame True {
              n217 = Replace Array Subset(array=w467, new element=w464, index=w466) -> (w465:T6[])
            }
          }
          n218 = Flatten To JSON(anything=w438) -> (JSON string=w437:string, 11:w436:errorcluster)  [unwired: 2 in]
          n219 = Write to Text File(file (use dialog)=w435, text=w437, error in=w436) -> (refnum out=w434:refnum<file>, error out=w433:errorcluster)  [unwired: 1 in, 1 out]
          n220 = Close File(refnum=w434, error in=w433) -> ()  [unwired: 2 out]
        }
        frame "Change Preset" {
          w494 = T6[] []
          n221 = Unbundle By Name(w488) -> ("Preset Index"=w486:i32)
          n222 = Read from Text File(file (use dialog)=w489) -> (refnum out=w493:refnum<file>, text=w490:string, error out=w492:errorcluster)  [unwired: 3 in, 1 out]
          n223 = Get Notifier Status(notifier=w474) -> (notifier out=w475:refnum<notifier>, current notification=w476:T4)  [unwired: 1 in, 3 out]
          n224 = Bundle By Name(cluster=w476, "Set Step"=0) -> (w477:T4)
          n225 = Close File(refnum=w493, error in=w492) -> (error out=w491:errorcluster)  [unwired: 1 out]
          n226 = Unflatten From JSON(JSON string=w490, type and defaults=w494, error in (no error)=w491) -> (value=w495:T6[], error out=w496:errorcluster)  [unwired: 4 in]
          n227 = Send Notification(notification=w477, notifier=w475) -> (notifier out=w472:refnum<notifier>)  [unwired: 1 in, 1 out]
          n228 = case shown="No Error" w496 {
            tunnel: w495 -> [w511 _]
            tunnel: w494 -> [_ w512]
            tunnel: [w511 w512] -> w487
            frame No Error {
            }
            frame Error {
            }
          }
          n229 = Index Array(array=w487, index=w486) -> (element=w485:T6)
          n230 = Unbundle By Name(w485) -> ("Steps"=w480:T7[])
          n231 = property on="Step" class="RadioBtnsControl (strict)"() -> ("Controls[]"=w482:refnum<vi>[])  [unwired: 2 in, 2 out]
          n232 = Array Size(array=w480) -> (size(s)=w479:i32)
          n233 = for {
            N: 5 -> [_]
            tunnel: w482 -> [w510] mode=indexing
            tunnel: w478 -> [w502] mode=indexing
            tunnel: w479 -> [w501]
            tunnel: w480 -> [w499] mode=indexing
            i -> [w507]
            w509 = refnum<vi> refnum  # Boolean
            n234 = Unbundle By Name(w499) -> ("Step Name"=w498:string)
            n235 = Increment(x=w507) -> (x+1=w506:i32)
            n236 = Less Or Equal?(x=w506, y=w501) -> (x <= y?=w505:bool)
            n237 = To More Specific Class(target class=w509, reference=w510) -> (specific class reference=w508:refnum<vi>)  [unwired: 1 in, 1 out]
            n238 = Select(t=T11."Enabled" ("Disabled"), s=w505, f=T11."Disabled and Grayed Out") -> (s? t:f=w500:T11)
            n239 = property class="Bool"(reference=w508, "BoolText.Text"=w498, "DisabledEnum"=w500) -> ()  [unwired: 1 in, 2 out]
            n240 = property class="Str"(reference=w502, "Value"=w498, "DisabledEnum"=w500) -> ()  [unwired: 1 in, 2 out]
          }
        }
        frame "Update Names" {
          n241 = property on="Step" class="RadioBtnsControl (strict)"() -> ("Controls[]"=w514:refnum<vi>[])  [unwired: 2 in, 2 out]
          n242 = Array Size(array=w516) -> (size(s)=w515:i32)
          n243 = for {
            N: w515 -> [_]
            tunnel: w516 -> [w526] mode=indexing
            tunnel: [w522] -> w517 mode=indexing
            tunnel: w514 -> [w521] mode=indexing
            w524 = refnum<vi> refnum  # Boolean
            n244 = To More Specific Class(target class=w524, reference=w521) -> (specific class reference=w525:refnum<vi>)  [unwired: 1 in, 1 out]
            n245 = property class="Bool"(reference=w525) -> ("BoolText.Text"=w523:string)  [unwired: 1 in, 2 out]
            n246 = Bundle By Name(cluster=w526, "Step Name"=w523) -> (w522:T7)
          }
        }
        frame "Quit" {
          n247 = Array Size(array=w531) -> (size(s)=w530:i32)
          n248 = Equal?(x=w533, y=w532) -> (x = y?=w528:bool)
          n249 = Equal To 0?(x=w530) -> (x = 0?=w529:bool)
          n250 = Or(x=w529, y=w528) -> (x .or. y?=w527:bool)
          n251 = Get Notifier Status(notifier=w535) -> (notifier out=w536:refnum<notifier>, current notification=w537:T4)  [unwired: 1 in, 3 out]
          n252 = Bundle By Name(cluster=w537, "Last Step?"=w527) -> (w538:T4)
          n253 = Send Notification(notification=w538, notifier=w536) -> (notifier out=w534:refnum<notifier>)  [unwired: 1 in, 1 out]
        }
      }
    }
    n254 = Get Notifier Status(notifier=w190) -> (notifier out=w194:refnum<notifier>, current notification=w193:T4)  [unwired: 1 in, 3 out]
    n255 = Bundle By Name(cluster=w193, "Received?"=TRUE) -> (w191:T4)
    n256 = Send Notification(notification=w191, notifier=w194) -> (notifier out=w189:refnum<notifier>)  [unwired: 1 in, 1 out]
  }
  n257 = To Word Integer(number=w82) -> (16bit integer=w84:i16)
  n258 = To Word Integer(number=w85) -> ()  [unwired: 1 out]
  n259 = property class="Bool (strict)"(reference=w69) -> ("Height"=w87:u32, "Top"=w88:i32)  [unwired: 1 in, 2 out]
  n260 = Unbundle By Name(w79) -> ("Left"=w81:i16, "Top"=w92:i16)
  n261 = To Word Integer(number=w87) -> (16bit integer=w90:i16)
  n262 = To Word Integer(number=w88) -> (16bit integer=w91:i16)
  n263 = Add(x=w81, y=w84) -> (x+y=w83:i16)
  n264 = Compound Arithmetic op=ADD(w92, w90, w91, i16 12 ("y")) -> (w86:i16)
  n265 = Bundle By Name(cluster=w79, "Right"=w83, "Bottom"=w86) -> (w80:T12)
  n266 = property class="VI"(reference=w78, "Front Panel.PanelBounds"=w80) -> ()  [unwired: 1 in, 2 out]
  n267 = local write "Quit"(w10) -> ()
  n268 = Release Notifier(notifier=w34, force destroy? (F)=TRUE) -> ()  [unwired: 1 in, 3 out]
